vi "kernel32_GetDriveTypeA.vi"(8 "错误输入（无错误）":errorcluster, 11 "lpRootPathName":string) -> (0 "错误输出":errorcluster, 3 "Type":T1(ring))   [LabVIEW 2011]
uses:
  kernel32.dll
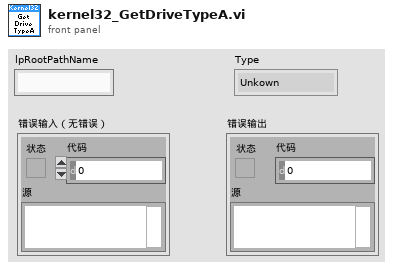
[diagram p1: front panel]
types:
  T1 = enum16{"Unkown", "No Root", "Removable", "Fixed", "Remote", "CD Rom", "Ramdisk"}
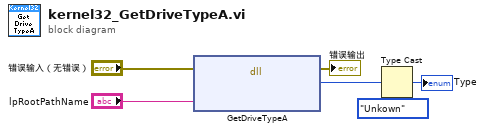
[diagram p0: block diagram]
diagram:
  n1 = dll-call lib="kernel32.dll" fn="GetDriveTypeA" ("GetDrive Type")(error in="错误输入（无错误）", "lpRootPathName"="lpRootPathName") -> (error out=→"错误输出":errorcluster, "返回类型"=w3:u16)  [unwired: 3 in, 1 out]
  n2 = Type Cast(type=T1."Unkown" ("Drive Type"), x=w3) -> (*(type *) &x=→"Type":T1)
